vi "Format Attribute Value String.vi"(8 "error in (no error)":errorcluster, 11 "Data":variant) -> (0 "error out":errorcluster, 3 "Value as String":string)   [LabVIEW 2020, in "XML.lvlib" / "XML.lvclass"]
uses:
  <vilib>/gpm_packages/@cs/persistence/source/XML/XML.lvclass
  <vilib>/Utility/Data Type/NI_Data Type.lvlib
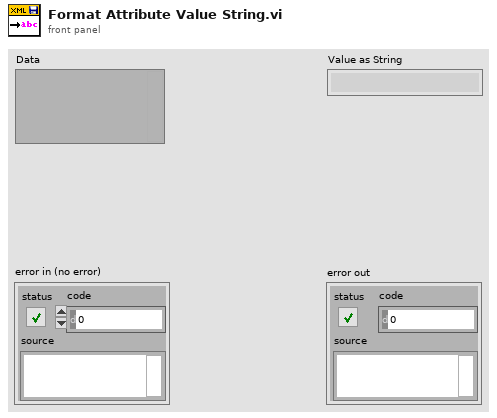
[diagram p1: front panel]
types:
  T1 = typedef "NI_Data Type.lvlib/Data Type.ctl" = enum8{"Invalid Type", "Void", "I8", "I16", "I32", "I64", "U8", "U16", "U32", "U64", "Single Float", "Double Float", "Extended Float", "Single Complex", "Double Complex", "Extended Complex", "Enum U8", "Enum U16", "Enum U32", "Enum U64", "Single Float With Unit", "Double Float With Unit", "Extended Float With Unit", "Single Complex with Unit", "Double Complex with Unit", "Extended Complex with Unit", "Boolean", "String", "Path", "Picture", "Tag", "Array", "Cluster", "Variant", "LV Variant", "Waveform", "Timestamp", "Digital Waveform", "Digital Data", "ExpressData", "Refnum", "External Data", "VI", "Poly VI", "LabVIEW Class Instance", "Fixed Point", "Set Collection", "Map Collection"}
  T2 = typedef "NI_Data Type.lvlib/VI Server Generic Type.ctl" = enum16{"NoType", "\tkLVObjApp=0x1", "\tkLVObjVI", "\tkLVObjGeneric", "\tkLVObjDecoration", "\tkLVObjText", "\tkLVObjControl", "\tkLVObjColorBox", "\tkLVObjBoolean", "\tkLVObjRefNum", "\tkLVObjVariant", "\tkLVObjPath", "\tkLVObjListBox", "\tkLVObjTable", "\tkLVObjArray", "\tkLVObjPicture", "\tkLVObjOleContainer", "\tkLVObjNumeric", "\tkLVObjDigital", "\tkLVObjNamedNumeric", "\tkLVObjColorRamp", "\tkLVObjSlide", "\tkLVObjGraphOrChart", "\tkLVObjWaveformChart", "\tkLVObjWaveformGraph", "\tkLVObjIntensityChart", "\tkLVObjIntensityGraph", "\tkLVObjString", "\tkLVObjIOName", "\tkLVObjComboBox", "\tkLVObjCluster", "\tkLVObjPanel", "\tkLVObjKnob", "\tkLVObjNumWithScale", "\tkLVObjRing", "\tkLVObjEnum", "\tkLVObjGObject", "\tkLVObjPlot", "\tkLVObjCursor", "\tkLVObjNumericText", "\tkLVObjScale", "\tkLVObjColorScale", "\tkLVObjGraphScale", "\tkLVObjColorGraphScale", "\tkLVObjTypedRefNum", "\tkLVObjOldKnobScale", "\tkLVObjMCListbox", "\tkLVObjMeasureData", "\tkLVObjDSCTag", "\tkLVObjDAQName", "\tkLVObjVISAName", "\tkLVObjIVIName", "\tkLVObjSlideScale", "\tkLVObjTabControl", "\tkLVObjPage", "\tkLVObjTabArrayTabControl", "\tkLVObjConPane", "\tkLVObjDAQMXName", "\tkLVObjVIRefNum", "\tkLVObjLVObjRefNum", "\tkLVObjAbsTime", "\tkLVObjDigitalTable", "\tkLVObjUnused", "\tkLVObjUnused2", "\tkLVObjSCLControl", "\tkLVObjSubPanel", "\tkLVObjTreeControl", "\tkLVObjGenClassTagRef", "\tkLVObjGenClassRef", "\tkLVObjRotaryColorScale", "\tkLVObjPlugInDDOControl", "\tkLVObjPlugInDDOClassHolder", "\tkLVObjRadClusControl", "\tkLVObjProject", "\tkLVObjProjectItem", "\tkLVObjPane", "\tkLVObjSplitterBar", "\tkLVObjProjectBuildItem", "\tkLVObjPixmap", "\tkLVObjFacadeVI", "\tkLVObjLibrary", "\tkLVObjVariable", "\tkLVObjPropertyBag", "\tkLVObjXYGraph", "\tkLVObjScene", "\tkLVObjUDClassLibrary", "\tkLVObjUDClassClone", "\tkLVObjMethodVI", "\tkLVObjXCtlLibrary", "\tkLVObjXNodeLibrary", "\tkLVObjScroll", "\tkLVObjLVTarget", "\tkLVObjMixedGraph", "\tkLVObjProvider", "\tkLVObjCopyOperation", "\tkLVObjTargetItem", "\tkLVObjProjectItemType", "\tkLVObjCopyItem", "\tkLVObjCopyConflict", "\tkLVObjCopyExpert", "\tkLVObjSceneGraphDisp", "\tkLVObjPolyVI", "\tkLVObjLVClassDDO", "kLVObjDiagram=0x4000", "\tkLVObjTerminal", "\tkLVObjConstant", "\tkLVObjPathConstant", "\tkLVObjArrayConstant", "\tkLVObjNumericConstant", "\tkLVObjDigitalNumConstant", "\tkLVObjNamedNumericConstant", "\tkLVObjStringConstant", "\tkLVObjClusterConstant", "\tkLVObjFixedConstant", "\tkLVObjControlTerminal", "\tkLVObjFormulaParameter", "\tkLVObjGlobal", "\tkLVObjLocal", "\tkLVObjRightShiftRegister", "\tkLVObjFunction", "\tkLVObjSubVI", "\tkLVObjCallByRef", "\tkLVObjUnitCast", "\tkLVObjStructure", "\tkLVObjLoop", "\tkLVObjMultiframeStructure", "\tkLVObjSequence", "\tkLVObjCaseSelector", "\tkLVObjFormula", "\tkLVObjGrowableFunction", "\tkLVObjBuildClusterArray", "\tkLVObjCompoundArithmetic", "\tkLVObjIndexArray", "\tkLVObjBuildArray", "\tkLVObjNamedBundler", "\tkLVObjCIN", "\tkLVObjCallLibrary", "\tkLVObjObjectFunction", "\tkLVObjProperty", "\tkLVObjInvoke", "\tkLVObjNode", "\tkLVObjBooleanConstant", "\tkLVObjBlockDiagram", "\tkLVObjRingConstant", "\tkLVObjEnumConstant", "\tkLVObjTunnel", "\tkLVObjLoopTunnel", "\tkLVObjSequenceLocal", "\tkLVObjComparison", "\tkLVObjReadWriteFile", "\tkLVObjTypeCast", "\tkLVObjFlattenUnflattenString", "\tkLVObjGPIBReadWrite", "\tkLVObjForLoop", "\tkLVObjWhileLoop", "\tkLVObjScriptNode", "\tkLVObjArrayToCluster", "\tkLVObjFormatScanString", "\tkLVObjWire", "\tkLVObjProbe", "\tkLVObjInnerTerminal", "\tkLVObjLeftShiftRegister", "\tkLVObjPolySubVI", "\tkLVObjPropItem", "\tkLVObjIONameConstant", "\tkLVObjDSCTagConstant", "\tkLVObjDAQNameConstant", "\tkLVObjVISANameConstant", "\tkLVObjIVINameConstant", "\tkLVObjColorBoxConstant", "\tkLVObjControlRefConstant", "\tkLVObjClassSpecifierConstant", "\tkLVObjConfNode", "\tkLVObjMasterWizard", "\tkLVObjStateDiagWizard", "\tkLVObjOuterTerminal", "\tkLVObjDAQMXNameConstant", "\tkLVObjEventStructure", "\tkLVObjFlatSequence", "\tkLVObjGenClassTagRefConstant", "\tkLVObjAbsTimeConstant", "\tkLVObjExternalNode", "\tkLVObjSubWizard", "\tkLVObjScriptNodeParameter", "\tkLVObjStatVIRef", "\tkLVObjComboBoxConstant", "\tkLVObjTimedLoop", "\tkLVObjGenClassDeepCopy", "\tkLVObjGenClassTagFlat", "\tkLVObjGenClassTagFlatRefConstant", "\tkLVObjGenClassFlat", "\tkLVObjSimDiagram", "\tkLVObjCompDiagram", "\tkLVObjSimNode", "\tkLVObjSimDCO", "\tkLVObjBundler", "\tkLVObjUnbundler", "\tkLVObjNamedUnbundler", "\tkLVObjFlatSeqFrame", "\tkLVObjFlatSeqInTun", "\tkLVObjFlatSeqOutTun", "\tkLVObjRefNumConst", "\tkLVObjFlattenString", "\tkLVObjPolySelector", "\tkLVObjXNode", "\tkLVObjSelectorTunnel", "\tkLVObjCommentNode", "\tkLVObjSdfDiagram", "\tkLVObjSDFCompDiagram", "\tkLVObjSdfNode", "\tkLVObjSdfDCO", "\tkLVObjFileDialog", "\tkLVObjTLDCO", "\tkLVObjTimeSeqFrame", "\tkLVObjTimeFlatSequence", "\tkLVObjTimedSequence", "\tkLVObjXDataNode", "\tkLVObjCodeWizard", "\tkLVObjMathScriptNode", "\tkLVObjMathScriptNodeParameter", "\tkLVObjLVClassBDConst"}
  T3 = typedef "NI_Data Type.lvlib/Refnum Type.ctl" = enum16{"NotARefnum", "UnknownRefnum", "Generic", "Datalog", "ByteStream", "Device", "Occurence", "TCPNetConnection", "Auto", "Menu", "Imaq", "Hardware", "DataSocket", "Visa", "IVI", "UDPNetConnection", "Notifier", "Queue", "Irda", "EventReg", "DotNet", "UserEvent", "Callback", "UNUSED_EMPTY_POSITION", "BlueToothNetConnection", "LVObjApp", "LVObjVI", "LVObjUnknown", "GenericClass", "UserDefinedRefnumTag", "DataValue", "RT FIFO", "TDMS File", "PythonSessionRefnum"}
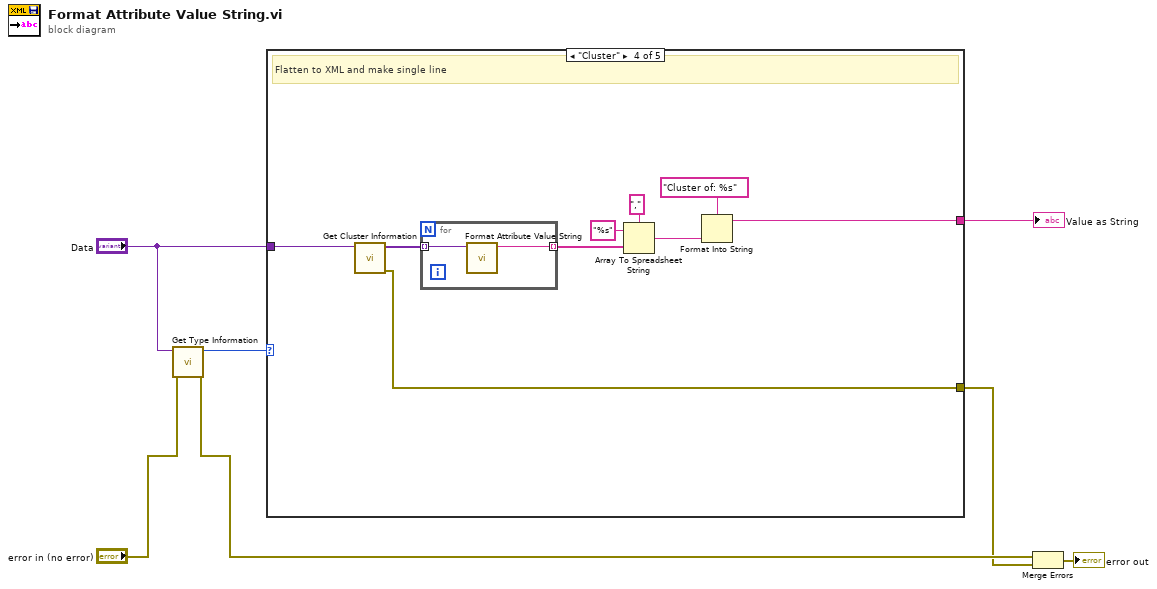
[diagram p0: block diagram]
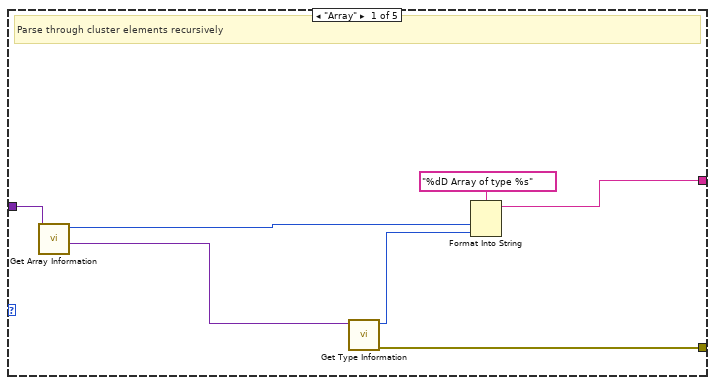
[diagram p2: hidden frame]
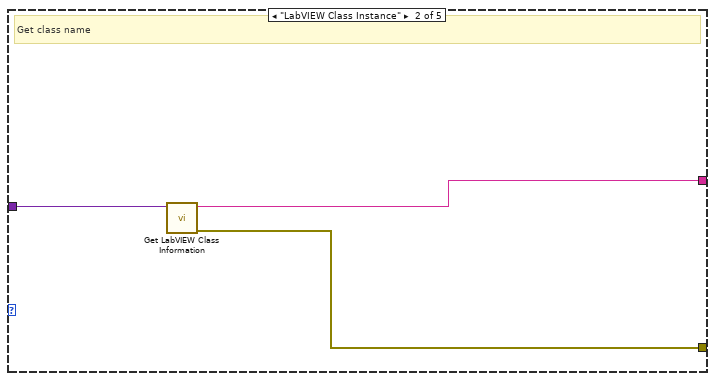
[diagram p3: hidden frame]
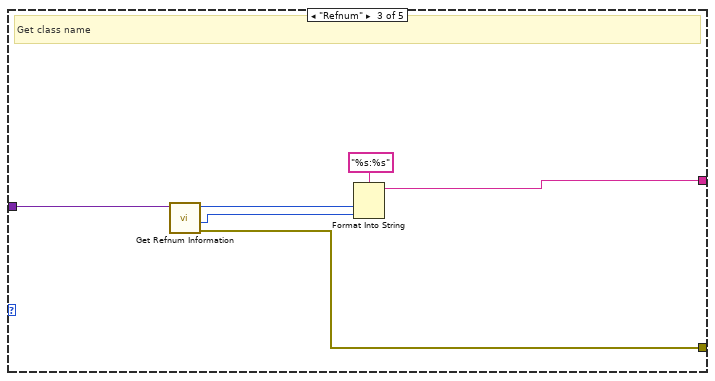
[diagram p4: hidden frame]
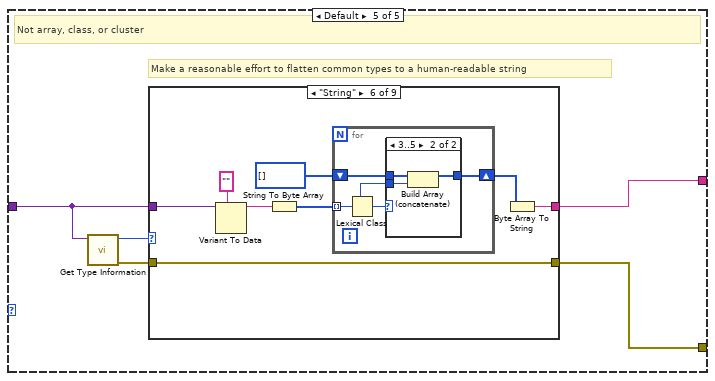
[diagram p5: hidden frame]
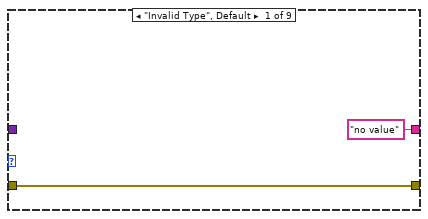
[diagram p6: hidden frame]
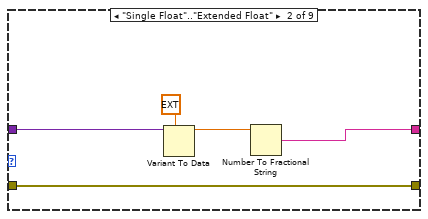
[diagram p7: hidden frame]
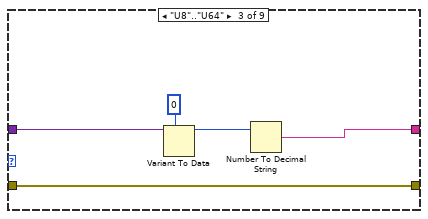
[diagram p8: hidden frame]
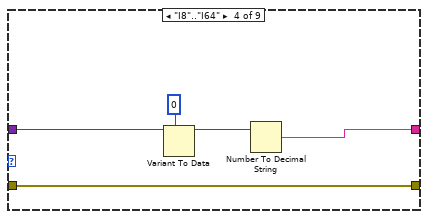
[diagram p9: hidden frame]
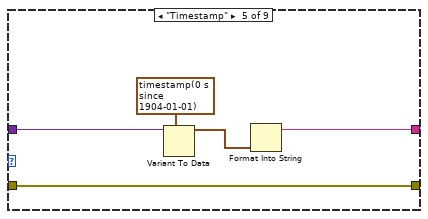
[diagram p10: hidden frame]
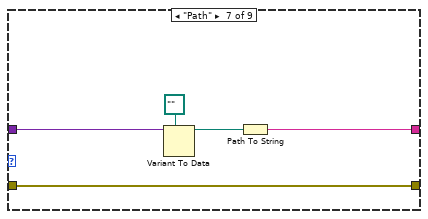
[diagram p12: hidden frame]
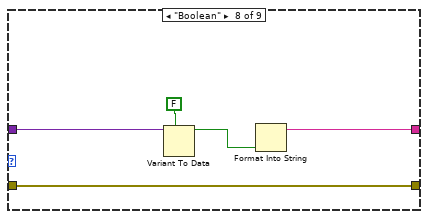
[diagram p13: hidden frame]
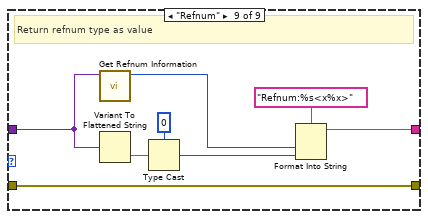
[diagram p14: hidden frame]
diagram:
  n1 = call <vilib>:"Get Type Information.vi"("error in (no error)"="error in (no error)", "variant"="Data") -> ("error out"=w4:errorcluster, "type"=w6:T1)  [unwired: 5 in, 3 out]
  n2 = case shown="\"Cluster\"" w6 {
    tunnel: [w14 w16 w18 w24 w36] -> w7
    tunnel: "Data" -> [w12 w17 w23 w32 w37]
    tunnel: [w13 w15 w22 w30 w35] -> w1
    frame "Array" {
      # "Parse through cluster elements recursively"
      n3 = call <vilib>:"Get Array Information.vi"("variant"=w12) -> ("array element data type"=w10:variant, "number of dimensions"=w11:i32)  [unwired: 7 in, 2 out]
      n4 = call <vilib>:"Get Type Information.vi"("variant"=w10) -> ("error out"=w13:errorcluster, "type"=w8:T1)  [unwired: 6 in, 3 out]
      n5 = Format Into String(format string="%dD Array of type %s", w11, w8) -> (resulting string=w14:string)  [unwired: 2 in, 1 out]
    }
    frame "LabVIEW Class Instance" {
      # "Get class name"
      n6 = call <vilib>:"Get LabVIEW Class Information.vi"("variant"=w17) -> ("error out"=w15:errorcluster, "LabVIEW class file name"=w16:string)  [unwired: 8 in, 1 out]
    }
    frame "Refnum" {
      # "Get class name"
      n7 = call <vilib>:"Get Refnum Information.vi"("variant"=w23) -> ("error out"=w22:errorcluster, "VI Server generic type"=w19:T2, "reference type"=w20:T3)  [unwired: 7 in, 1 out]
      n8 = Format Into String(format string="%s:%s", w20, w19) -> (resulting string=w18:string)  [unwired: 2 in, 1 out]
    }
    frame "Cluster" {
      # "Flatten to XML and make single line"
      n9 = call <vilib>:"Get Cluster Information.vi"("variant"=w32) -> ("error out"=w30:errorcluster, "cluster elements"=w31:variant[])  [unwired: 9 in]
      n10 = for {
        tunnel: w31 -> [w34] mode=indexing
        tunnel: [w33] -> w29 mode=indexing
        n11 = call <vilib>:"Format Attribute Value String.vi"("Data"=w34) -> ("Value as String"=w33:string)  [unwired: 9 in, 1 out]
      }
      n12 = Array To Spreadsheet String(delimiter (Tab)=",", array=w29, 3:"%s" ("format string")) -> (spreadsheet string=w26:string)
      n13 = Format Into String(format string="Cluster of: %s", w26) -> (resulting string=w24:string)  [unwired: 2 in, 1 out]
    }
    frame Default {
      # "Make a reasonable effort to flatten common types to a human-readable string"
      # "Not array, class, or cluster"
      n14 = call <vilib>:"Get Type Information.vi"("variant"=w37) -> ("error out"=w39:errorcluster, "type"=w38:T1)  [unwired: 6 in, 3 out]
      n15 = case shown="\"String\"" w38 {
        tunnel: w37 -> [_ w45 w50 w55 w60 w68 w81 w86 w91]
        tunnel: ["no value" w44 w49 w54 w57 w63 w79 w83 w93] -> w36
        tunnel: w39 -> [w41 w42 w47 w52 w59 w67 w78 w85 w95]
        tunnel: [w41 w42 w47 w52 w59 w67 w78 w85 w95] -> w35
        frame "Invalid Type", Default {
        }
        frame "Single Float".."Extended Float" {
          n16 = Variant To Data(type=ext 0.0, Variant=w45) -> (data=w43:ext)  [unwired: 1 in, 1 out]
          n17 = Number To Fractional String(number=w43) -> (F-format string=w44:string)  [unwired: 3 in]
        }
        frame "U8".."U64" {
          n18 = Variant To Data(type=u64 0, Variant=w50) -> (data=w48:u64)  [unwired: 1 in, 1 out]
          n19 = Number To Decimal String(number=w48) -> (decimal integer string=w49:string)  [unwired: 1 in]
        }
        frame "I8".."I64" {
          n20 = Variant To Data(type=i64 0, Variant=w55) -> (data=w53:i64)  [unwired: 1 in, 1 out]
          n21 = Number To Decimal String(number=w53) -> (decimal integer string=w54:string)  [unwired: 1 in]
        }
        frame "Timestamp" {
          n22 = Variant To Data(type=timestamp(0 s since 1904-01-01), Variant=w60) -> (data=w58:timestamp)  [unwired: 1 in, 1 out]
          n23 = Format Into String(w58) -> (resulting string=w57:string)  [unwired: 3 in, 1 out]
        }
        frame "String" {
          n24 = Variant To Data(type="", Variant=w68) -> (data=w66:string)  [unwired: 1 in, 1 out]
          n25 = String To Byte Array(string=w66) -> (unsigned byte array=w65:u8[])
          n26 = for {
            tunnel: w65 -> [w72] mode=indexing
            shift-right: [w71] -> w62
            shift-left: u8[] [] ("unsigned byte array") -> [w70]
            n27 = Lexical Class(1:w72) -> (0:w73:i16)
            n28 = case shown="3..5" w73 {
              tunnel: w72 -> [_ w77]
              tunnel: [w74 w75] -> w71
              tunnel: w70 -> [w74 w76]
              frame Default {
              }
              frame 3..5 {
                n29 = Build Array (concatenate)(w76, w77) -> (w75:u8[])
              }
            }
          }
          n30 = Byte Array To String(unsigned byte array=w62) -> (string=w63:string)
        }
        frame "Path" {
          n31 = Variant To Data(type=path "", Variant=w81) -> (data=w80:path)  [unwired: 1 in, 1 out]
          n32 = Path To String(path=w80) -> (string=w79:string)
        }
        frame "Boolean" {
          n33 = Variant To Data(type=FALSE, Variant=w86) -> (data=w84:bool)  [unwired: 1 in, 1 out]
          n34 = Format Into String(w84) -> (resulting string=w83:string)  [unwired: 3 in, 1 out]
        }
        frame "Refnum" {
          # "Return refnum type as value"
          n35 = call <vilib>:"Get Refnum Information.vi"("variant"=w91) -> ("reference type"=w94:T3)  [unwired: 7 in, 3 out]
          n36 = Variant To Flattened String(Variant=w91) -> (data string=w90:string)  [unwired: 1 out]
          n37 = Type Cast(type=u32 0, x=w90) -> (*(type *) &x=w88:u32)
          n38 = Format Into String(format string="Refnum:%s<x%x>", w94, w88) -> (resulting string=w93:string)  [unwired: 2 in, 1 out]
        }
      }
    }
  }
  "Value as String" <- w7
  n39 = Merge Errors(w4, w1) -> (→"error out":errorcluster)
